vi "MAVLink GPS POS.vi"(7 "FGV Method":T2, 11 "Position":T1) -> (3 "Position out":T1)   [LabVIEW 2014]
uses:
  Controls/FGV Methods.ctl
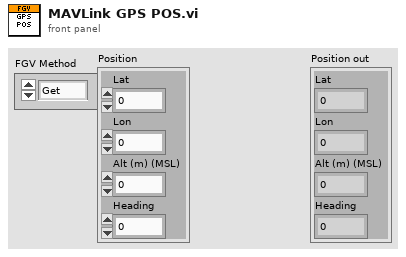
[diagram p1: front panel]
types:
  T1 = cluster{"Lat":sgl, "Lon":sgl, "Alt (m) (MSL)":sgl, "Heading":dbl}
  T2 = typedef "FGV Methods.ctl" = enum16{"Get", "Set"}
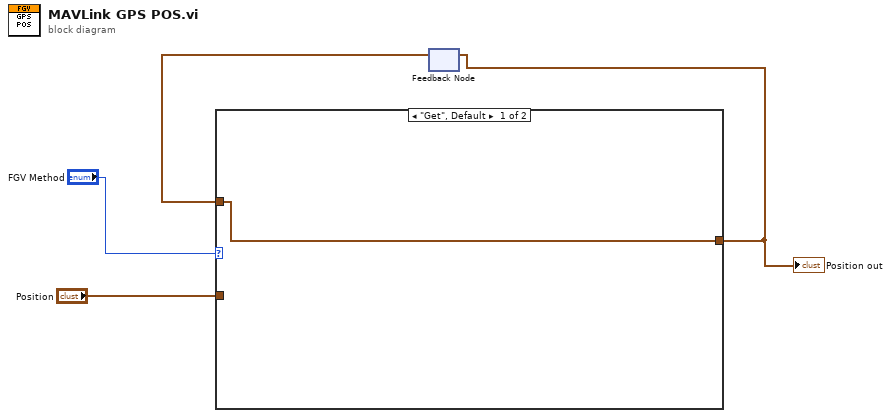
[diagram p0: block diagram]
diagram:
  n1 = feedback #1() -> (w2:T1)  [unwired: 1 in]
  n2 = case shown="\"Get\", Default" "FGV Method" {
    tunnel: "Position" -> [_ w6]
    tunnel: [w5 w6] -> w3
    tunnel: w2 -> [w5 _]
    frame "Get", Default {
    }
    frame "Set" {
    }
  }
  "Position out" <- w3
  n3 = feedback-in #1(w3) -> ()
